vi "generatePressureSequence.vi"(7 "Set Pressures List":dbl[][](array[numeric])=[[665.1538332158755, 622.4106177021335]], 9 "Calibration Refs":T1, 10 "Ratio":dbl[](array[numeric])=[0.6, 0.6, 0.6, 0.6, 0.6, 0.6, 0.6, 0.6], 11 "Mix":u16[](array[ring])=[0, 0] items=["A1"=0, "A2"=1, "A3"=2, "A4"=3, "A5"=12]) -> (0 "error out":errorcluster, 1 "Missing Ratio":dbl[](array[numeric]), 2 "Missing Mix Valve":u16[](array[ring]) items=["A1"=0, "A2"=1, "A3"=2, "A4"=3, "A5"=12], 3 "Pressure For Mix":dbl[](array[numeric]), 5 "All Cal Data Missing?":bool)   [LabVIEW 2016]
uses:
  <vilib>/Utility/error.llb/Error Cluster From Error Code.vi
  <vilib>/ErrorRing/Error Ring.xnode
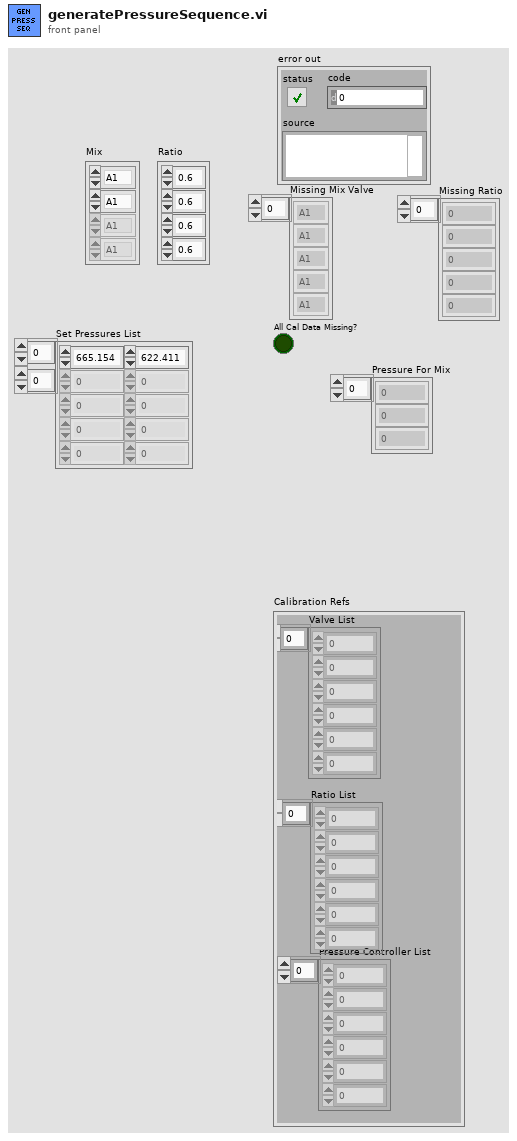
[diagram p1: front panel]
types:
  T1 = cluster{"Pressure Controller List":u8[], "Ratio List":dbl[], "Valve List":u16[]}
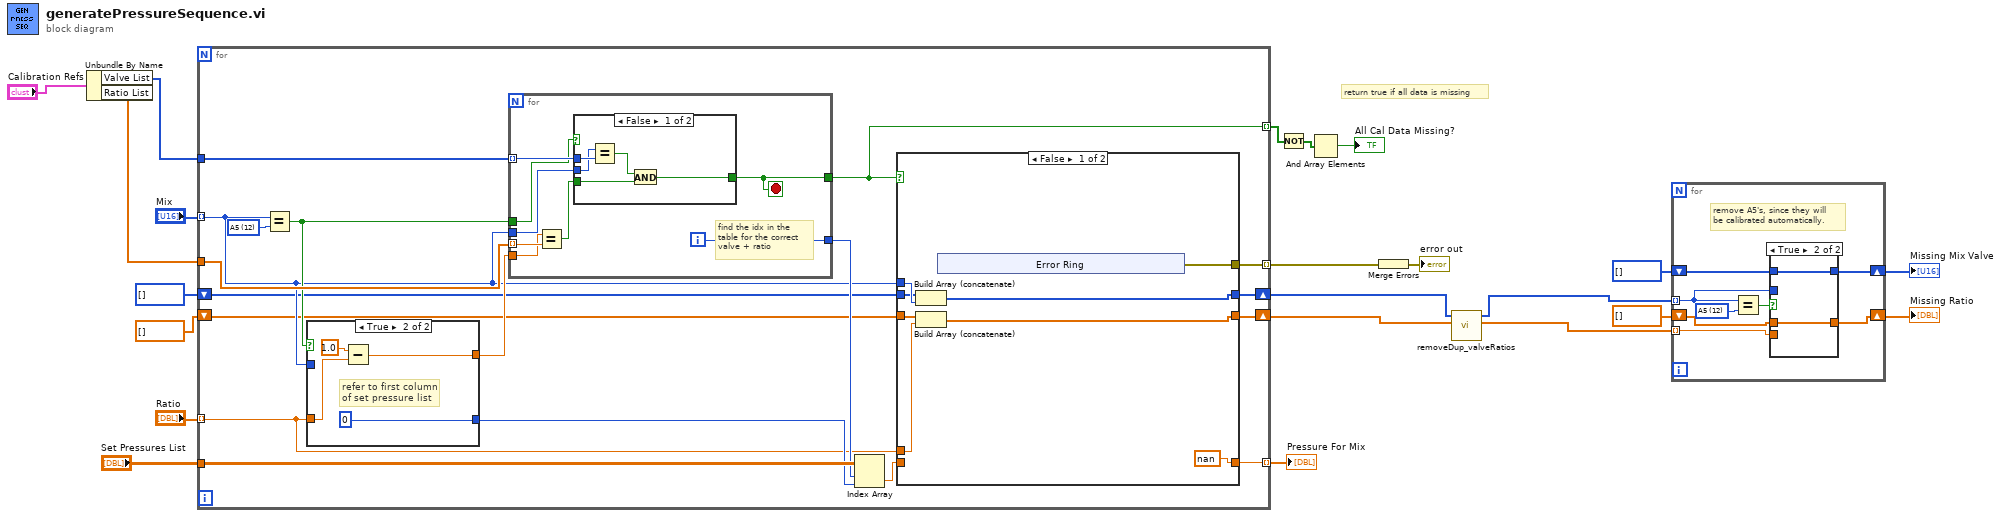
[diagram p0: block diagram]
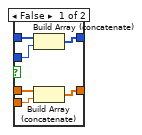
[diagram p2: hidden frame]
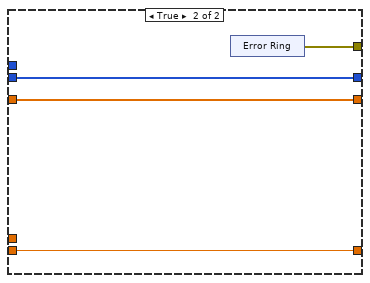
[diagram p3: hidden frame]
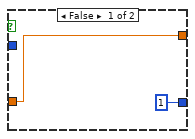
[diagram p5: hidden frame]
diagram:
  # "return true if all data is missing"
  n1 = Unbundle By Name("Calibration Refs") -> ("Valve List"=w2:u16[], "Ratio List"=w1:dbl[])
  n2 = for {
    tunnel: "Mix" -> [w29] mode=indexing
    tunnel: "Ratio" -> [w28] mode=indexing
    tunnel: w1 -> [w39]
    tunnel: w2 -> [w38]
    tunnel: "Set Pressures List" -> [w35]
    tunnel: [w31] -> w19 mode=indexing
    tunnel: [w30] -> w18 mode=indexing
    shift-right: [w26] -> w6
    shift-left: dbl[] [] -> [w27]
    shift-right: [w24] -> w7
    shift-left: u16[] [] -> [w25]
    tunnel: [w23] -> w10 mode=indexing
    w40 = u16 12 items=["A1"=0, "A2"=1, "A3"=2, "A4"=3, "A5"=12] ("Ring")
    n3 = Equal?(x=w29, y=w40) -> (x = y?=w36:bool)
    n4 = case shown="True" w36 {
      tunnel: w29 -> [_ _]
      tunnel: w28 -> [w73 w76]
      tunnel: [1 0] -> w33
      tunnel: [w73 w75] -> w37
      frame False {
      }
      frame True {
        # "refer to first column \nof set pressure list"
        n5 = Subtract(x=1.0, y=w76) -> (x-y=w75:dbl)
      }
    }
    n6 = for {
      tunnel: w39 -> [w64] mode=indexing
      tunnel: w38 -> [w66] mode=indexing
      tunnel: w29 -> [w65]
      tunnel: w37 -> [w63]
      tunnel: [w61] -> w34
      tunnel: [w60] -> w23
      tunnel: w36 -> [w59]
      i -> [w61]
      stop <- w60 stop-if-true
      # "find the idx in the\ntable for the correct\nvalve + ratio"
      n7 = Equal?(x=w63, y=w64) -> (x = y?=w62:bool)
      n8 = case shown="False" w59 {
        tunnel: w66 -> [w71 _]
        tunnel: w65 -> [w70 _]
        tunnel: w62 -> [w68 w72]
        tunnel: [w67 w72] -> w60
        frame False {
          n9 = Equal?(x=w70, y=w71) -> (x = y?=w69:bool)
          n10 = And(x=w69, y=w68) -> (x .and. y?=w67:bool)
        }
        frame True {
          # "for A5, don't care \nwhat the other valve was"
        }
      }
    }
    n11 = Index Array(array=w35, index (row)=w34, index (col)=w33) -> (element=w32:dbl)
    n12 = case shown="False" w23 {
      tunnel: [w48 w57] -> w30
      tunnel: w32 -> [_ w56]
      tunnel: [nan ("output") w56] -> w31
      tunnel: w29 -> [w43 _]
      tunnel: w28 -> [w46 _]
      tunnel: w27 -> [w45 w55]
      tunnel: [w44 w55] -> w26
      tunnel: w25 -> [w42 w54]
      tunnel: [w41 w54] -> w24
      frame False {
        n13 = Build Array (concatenate)(w42, w43) -> (w41:u16[])
        n14 = Build Array (concatenate)(w45, w46) -> (w44:dbl[])
        n15 = xnode "Error Ring"() -> ("error out"=w48:errorcluster)
      }
      frame True {
        n16 = xnode "Error Ring"() -> ("error out"=w57:errorcluster)
      }
    }
  }
  "Pressure For Mix" <- w19
  n17 = Not(x=w10) -> (.not. x?=w9:bool[])
  n18 = And Array Elements(Boolean array=w9) -> (logical AND=→"All Cal Data Missing?":bool)
  n19 = Merge Errors(w18) -> (→"error out":errorcluster)
  n20 = call "removeDup_valveRatios.vi"("Ratios"=w6, "Valves"=w7) -> ("Ratio with Dup Removed"=w4:dbl[], "Valves with Dup Removed"=w5:u16[])  [unwired: 8 in]
  n21 = for {
    tunnel: w5 -> [w80] mode=indexing
    tunnel: w4 -> [w85] mode=indexing
    shift-right: [w86] -> w12
    shift-left: u16[] [] -> [w82]
    shift-right: [w84] -> w11
    shift-left: dbl[] [] -> [w83]
    w81 = u16 12 items=["A1"=0, "A2"=1, "A3"=2, "A4"=3, "A5"=12] ("Ring")
    # "remove A5's, since they will \nbe calibrated automatically."
    n22 = Equal?(x=w80, y=w81) -> (x = y?=w79:bool)
    n23 = case shown="True" w79 {
      tunnel: w80 -> [w92 _]
      tunnel: [w91 w93] -> w86
      tunnel: w85 -> [w90 _]
      tunnel: [w89 w94] -> w84
      tunnel: w83 -> [w88 w94]
      tunnel: w82 -> [w87 w93]
      frame False {
        n24 = Build Array (concatenate)(w87, w92) -> (w91:u16[])
        n25 = Build Array (concatenate)(w88, w90) -> (w89:dbl[])
      }
      frame True {
      }
    }
  }
  "Missing Mix Valve" <- w12
  "Missing Ratio" <- w11
